vi "IT6724C_Config_Link.vi"(8 "error in":errorcluster caption="错误输入（无错误）", 10 "等待时间(毫秒)":u32=100, 11 "MyIndex":u8) -> (0 "error out":errorcluster, 3 "返回值":string)   [LabVIEW 2015, in "IT6724.lvlib"]
uses:
  IT6724.lvlib
  <vilib>/Instr/_visa.llb/VISA Configure Serial Port (Instr).vi
panel:
  out "VISA":refnum<visa-resource-name>
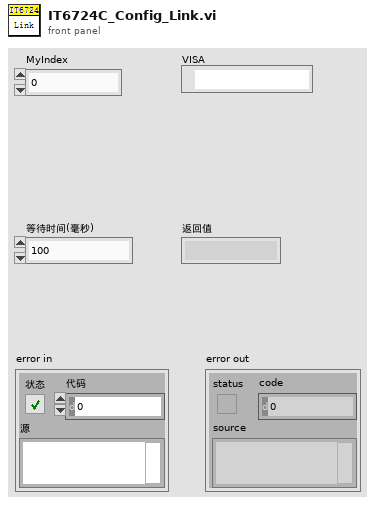
[diagram p1: front panel]
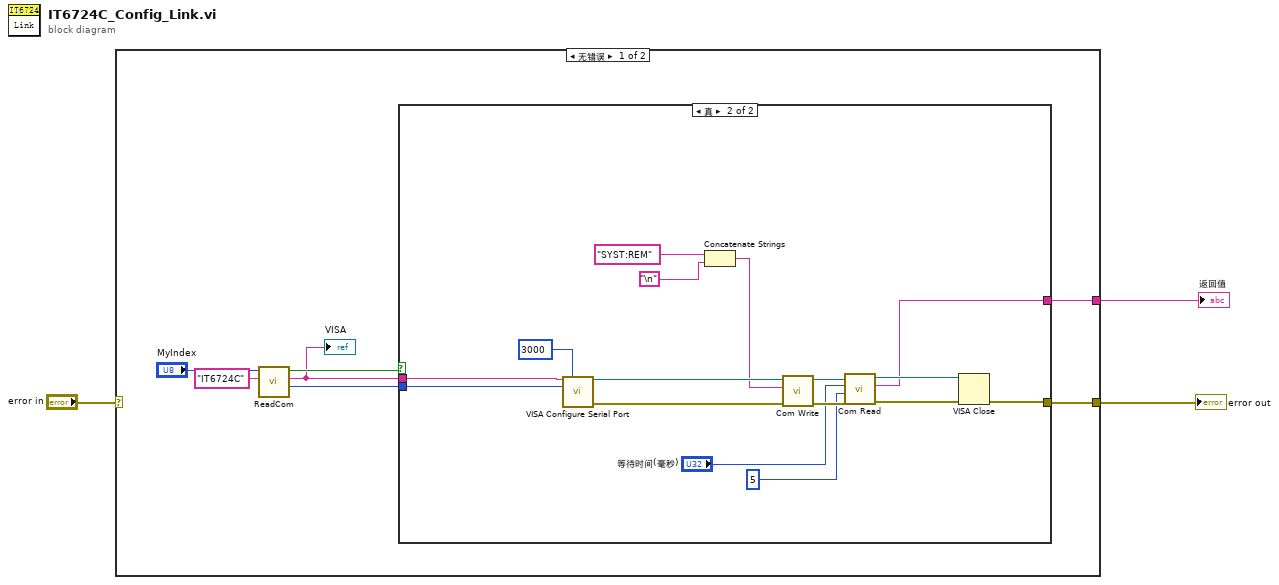
[diagram p0: block diagram]
diagram:
  n1 = case shown="无错误" "error in" {
    selector: "error in" -> [_ w27]
    tunnel: [w10 w27] -> w3
    tunnel: [w4 _] -> w1
    frame No Error {
      n2 = call "ReadCom.vi"("仪器名称"="IT6724C", "MyIndex"="MyIndex") -> ("Baudrate"=w5:i32, "COM"=w6:string, "OK?"=w7:bool)  [unwired: 7 in]
      "VISA" <- w6
      n3 = case shown="真" w7 {
        tunnel: [_ w26] -> w10
        tunnel: w6 -> [_ w25]
        tunnel: w5 -> [_ w24]
        tunnel: [_ w16] -> w4
        frame False {
        }
        frame True {
          n4 = call-poly "VISA Configure Serial Port"("VISA resource name"=w25, "timeout (10sec)"=u32 3000, "baud rate (9600)"=w24) -> ("VISA resource name out"=w22:refnum<visa-resource-name>, "error out"=w21:errorcluster)  [unwired: 11 in]
          n5 = Concatenate Strings("SYST:REM", "\n") -> (w14:string)
          n6 = call "Com Write.vi"("错误输入（无错误）"=w21, "Wbuff"=w14, "VISA In"=w22) -> ("错误输出"=w19:errorcluster, "VISA Out"=w20:refnum<visa-resource-name>)  [unwired: 7 in]
          n7 = call "Com Read.vi"("错误输入（无错误）"=w19, "num"=u32 5, "超时"="等待时间(毫秒)", "VISA In"=w20) -> ("错误输出"=w18:errorcluster, "buff"=w16:string, "VISA Out"=w17:refnum<visa-resource-name>)  [unwired: 5 in]
          n8 = VISA Close(VISA resource name=w17, error in (no error)=w18) -> (error out=w26:errorcluster)
        }
      }
    }
    frame Error {
    }
  }
  "error out" <- w3
  "返回值" <- w1
